vi "DDC Stage 02 - 1ch.vi"(1 "acq.reset":bool, 5 "ddc.out.rate":fxp<+,48,1>[](array[numeric])=[0.0, 0.0, 0.0, 0.0, 0.0, 0.0, 0.0, 0.0, 0.0, 0.0, 0.0, 0.0, 0.0, 0.0, 0.0, 0.0] format="%.48g", 7 "ddc.delay":fxp<+/-,16,0>[](array[numeric])=[0.0, 0.0, 0.0, 0.0, 0.0, 0.0, 0.0, 0.0, 0.0, 0.0, 0.0, 0.0, 0.0, 0.0, 0.0, 0.0] format="%.16g") -> (3 "dsp.overflow":bool, 6 "16xU32":u32[](array[numeric]), 10 "output valid":bool, 14 "dbg,output1":T1)   [LabVIEW 2015, in "DDC_7976R_v1.lvlib"]
uses:
  DDC_7976R_v1.lvlib
  Private/Typedef - internal -03.ctl
  Private/Typedef - internal -04.ctl
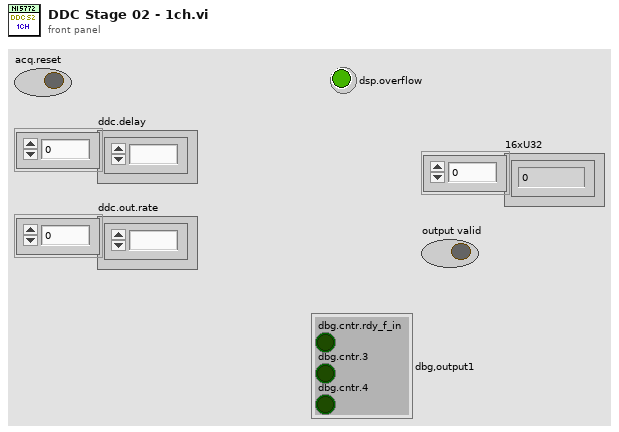
[diagram p1: front panel]
types:
  T1 = typedef "DDC_7976R_v1.lvlib/Typedef - internal -03.ctl" = cluster{"dbg.cntr.4":bool, "dbg.cntr.3":bool, "dbg.cntr.rdy_f_in":bool}
  T2 = typedef "DDC_7976R_v1.lvlib/Typedef - internal -04.ctl" = cluster{"acq.reset":bool, "ddc.out.rate":fxp<+,48,1>[], "ddc.delay":fxp<+/-,16,0>[], "Channel#":u8}
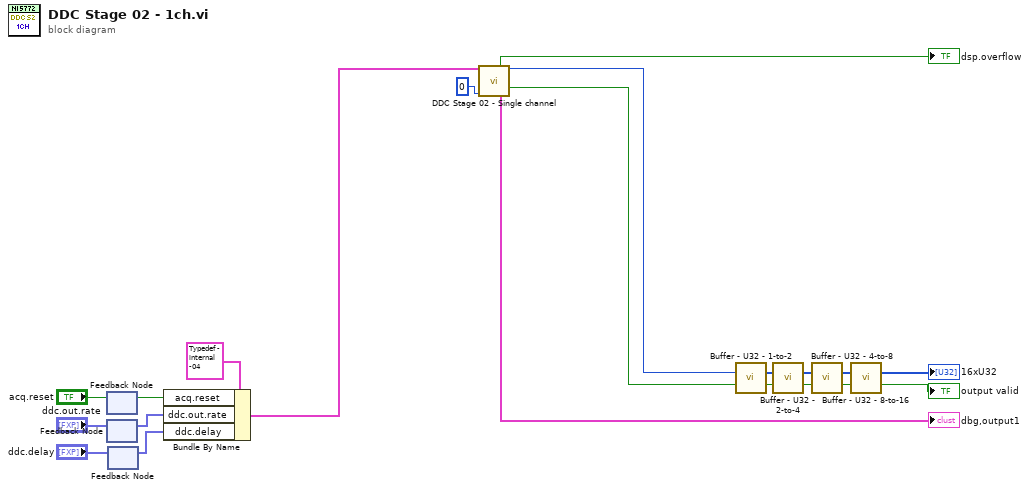
[diagram p0: block diagram]
diagram:
  n1 = feedback #1() -> (w15:bool)  [unwired: 1 in]
  n2 = feedback-in #1("acq.reset") -> ()
  n3 = feedback #2() -> (w16:fxp<+,48,1>[])  [unwired: 1 in]
  n4 = feedback-in #2("ddc.out.rate") -> ()
  n5 = feedback #3() -> (w1:fxp<+/-,16,0>[])  [unwired: 1 in]
  n6 = feedback-in #3("ddc.delay") -> ()
  n7 = Bundle By Name(cluster=T2 {"acq.reset"=FALSE, "ddc.out.rate"=[0.0, 0.0, 0.0, 0.0, 0.0, 0.0, 0.0, 0.0, 0.0, 0.0, 0.0, 0.0, 0.0, 0.0, 0.0, 0.0], "ddc.delay"=[0.0, 0.0, 0.0, 0.0, 0.0, 0.0, 0.0, 0.0, 0.0, 0.0, 0.0, 0.0, 0.0, 0.0, 0.0, 0.0], "Channel#"=0} ("output cluster 2"), "acq.reset"=w15, "ddc.out.rate"=w16, "ddc.delay"=w1) -> (w14:T2)
  n8 = call "DDC Stage 02 - Single channel.vi"("input cluster"=w14, "Ch#"=u8 0) -> ("dsp.overflow"=→"dsp.overflow":bool, "U32 out"=w4:u32, "output valid"=w3:bool, "dbg,output1"=→"dbg,output1":T1)  [unwired: 10 in]
  n9 = call "Buffer - U32 - 1-to-2.vi"("U32 in"=w4, "Input valid"=w3) -> ("Array 2 out"=w11:u32[], "Output valid"=w8:bool)  [unwired: 12 in]
  n10 = call "Buffer - U32 - 2-to-4.vi"("Array 2 in"=w11, "Input valid"=w8) -> ("Array4 out"=w10:u32[], "Output valid"=w7:bool)  [unwired: 12 in]
  n11 = call "Buffer - U32 - 4-to-8.vi"("Array4in"=w10, "Input valid"=w7) -> ("Array8 out"=w9:u32[], "Output valid"=w6:bool)  [unwired: 12 in]
  n12 = call "Buffer - U32 - 8-to-16.vi"("Array 8 in"=w9, "Input valid"=w6) -> ("Array 16 out"=→"16xU32":u32[], "Output valid"=→"output valid":bool)  [unwired: 12 in]
